vi "DLU.Next Node.vi"(2 "NumNodes":u8, 5 "Current Node":u8, 9 "Move to Next Node":bool) -> (6 "Next Node":u8)   [LabVIEW 2014, in "IO Node Logic Template_SPIBus0.lvlib"]
uses:
  IO Node Logic Template_SPIBus0.lvlib
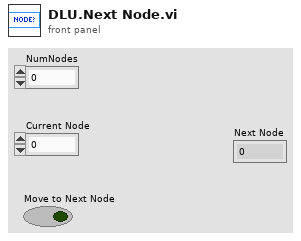
[diagram p1: front panel]
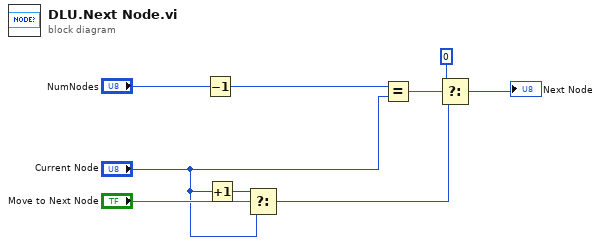
[diagram p0: block diagram]
diagram:
  n1 = Decrement(x="NumNodes") -> (x-1=w9:u8)
  n2 = Increment(x="Current Node") -> (x+1=w2:u8)
  n3 = Select(t=w2, s="Move to Next Node", f="Current Node") -> (s? t:f=w3:u8)
  n4 = Equal?(x=w9, y="Current Node") -> (x = y?=w5:bool)
  n5 = Select(t=u8 0, s=w5, f=w3) -> (s? t:f=→"Next Node":u8)
